vi "sum-of-array.vi"(1 "Array":dbl[](array[numeric])) -> (0 "sum of array":dbl)   [LabVIEW 2023]
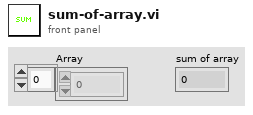
[diagram p1: front panel]
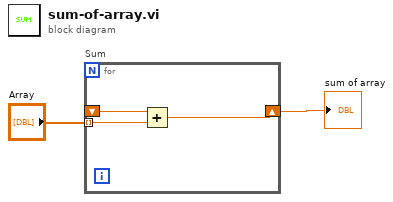
[diagram p0: block diagram]
diagram:
  n1 = for "Sum" {
    shift-right: [w4] -> w2
    shift-left: _ -> [w5]
    tunnel: "Array" -> [w3] mode=indexing
    n2 = Add(x=w5, y=w3) -> (x+y=w4:dbl)
  }
  "sum of array" <- w2
